vi "List Local Chassis Modules.vi"(8 "error in (no error)":errorcluster, 11 "Item Ref in":T1 format="%.0x") -> (0 "error out":errorcluster, 2 "Local Slots #":u32[](array[numeric]), 3 "Item Ref out":T1 format="%.0x")   [LabVIEW 2017, in "Scan Engine Custom Device.lvlib"]
doc: "This VI lists the module(s) configured in Local Chassis. GUIDs are used to create the list. The output is a list of Slot Number."
uses:
  Scan Engine Custom Device.lvlib
  <vilib>/NI Veristand/Custom Device API/Custom Device Item Ref.ctl
  Globals/Scan Engine GUIDs.vi
  <vilib>/NI Veristand/Custom Device Tools/Custom Device Utility Library/NI VeriStand - Search for Item by GUID.vi
  <vilib>/NI Veristand/Custom Device Tools/Custom Device Utility Library/Custom Device Utility Library.lvlib
  Modules.lvlibp/RSI Module/RSI Module.lvclass
  <vilib>/NI Veristand/Custom Device API/Custom Device API.lvlib
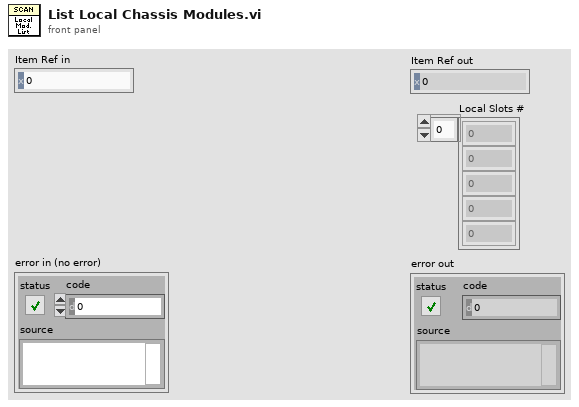
[diagram p1: front panel]
types:
  T1 = typedef "Custom Device API.lvlib/Custom Device Item Ref.ctl" = u64
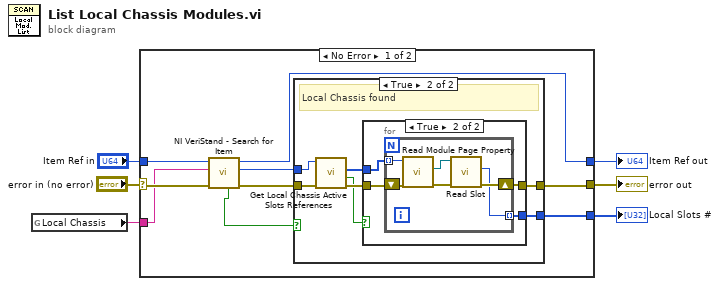
[diagram p0: block diagram]
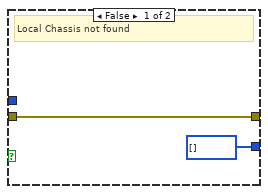
[diagram p2: hidden frame]
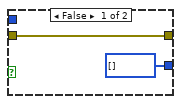
[diagram p3: hidden frame]
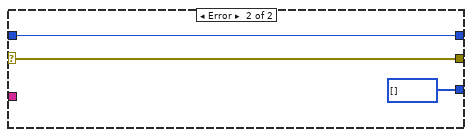
[diagram p4: hidden frame]
diagram:
  n1 = global read "Scan Engine GUIDs.vi" "Local Chassis"() -> (w3:string)
  n2 = case shown="No Error" "error in (no error)" {
    selector: "error in (no error)" -> [w15 w39]
    tunnel: [w8 w39] -> w5
    tunnel: "Item Ref in" -> [w14 w38]
    tunnel: w3 -> [w13 _]
    tunnel: [w9 w38] -> w2
    tunnel: [w7 u32[] []] -> w1
    frame No Error {
      n3 = call-poly <vilib>:"NI VeriStand - Search for Item.vi"("error in"=w15, "Item GUID"=w13, "Section Ref in"=w14) -> ("error out"=w11:errorcluster, "Item Ref"=w10:T1, "Section Ref out"=w9:T1, "Found"=w12:bool)  [unwired: 5 in]
      n4 = case shown="True" w12 {
        tunnel: w11 -> [w16 w24]
        tunnel: w10 -> [_ w23]
        tunnel: [w16 w21] -> w8
        tunnel: [u32[] [] w20] -> w7
        frame False {
          # "Local Chassis not found"
        }
        frame True {
          # "Local Chassis found"
          n5 = call "Get Local Chassis Active Slots References.vi"("error in"=w24, "Local Chassis Reference In"=w23) -> ("error out"=w22:errorcluster, "Modules Found"=w18:bool, "Slots References"=w19:T1[])  [unwired: 6 in, 1 out]
          n6 = case shown="True" w18 {
            tunnel: w22 -> [w26 w30]
            tunnel: [w26 w28] -> w21
            tunnel: w19 -> [_ w29]
            tunnel: [u32[] [] w27] -> w20
            frame False {
            }
            frame True {
              n7 = for {
                tunnel: w29 -> [w33] mode=indexing
                shift-right: [w32] -> w28
                shift-left: w30 -> [w36]
                tunnel: [w31] -> w27 mode=indexing
                n8 = call "Read Module Page Property.vi"("error in (no error)"=w36, "Node Ptr In"=w33) -> ("error out"=w35:errorcluster, "RSI Module"=w34:refnum<class "RSI Module.lvclass">)  [unwired: 7 in, 1 out]
                n9 = call "Read Slot.vi"("error in (no error)"=w35, "RSI Module in"=w34) -> ("error out"=w32:errorcluster, "Slot"=w31:u32)  [unwired: 7 in, 1 out]
              }
            }
          }
        }
      }
    }
    frame Error {
    }
  }
  "Item Ref out" <- w2
  "error out" <- w5
  "Local Slots #" <- w1
